vi "Time.Compare New Time with From_To to get new From_To Time Range.vi"(8 "Init":bool, 9 "PrevTo":timestamp, 10 "PrevFrom":timestamp, 11 "Start":timestamp) -> (1 "NewTo":timestamp, 2 "NewFrom":timestamp)   [LabVIEW 2019]
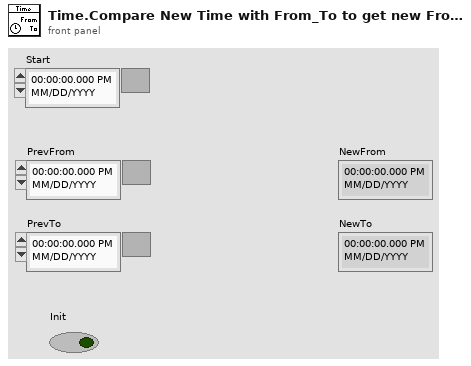
[diagram p1: front panel]
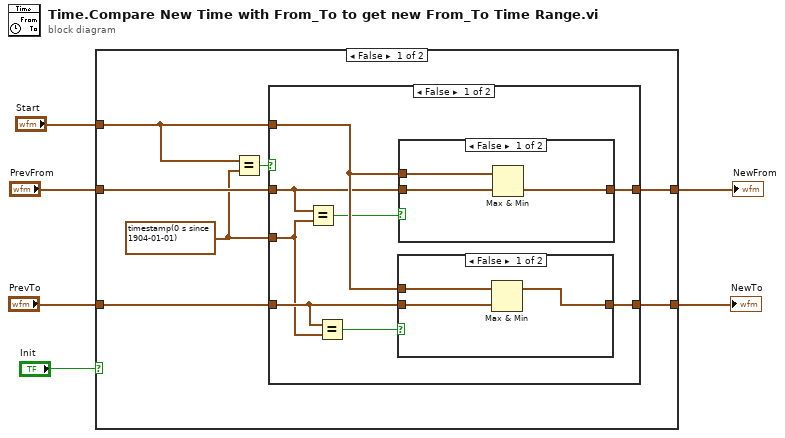
[diagram p0: block diagram]
diagram:
  n1 = case shown="False" "Init" {
    tunnel: "PrevFrom" -> [w13 _]
    tunnel: [w12 w32] -> w5
    tunnel: "Start" -> [w11 w32]
    tunnel: "PrevTo" -> [w9 _]
    tunnel: [w7 w32] -> w2
    frame False {
      w8 = timestamp(0 s since 1904-01-01)
      n2 = Equal?(x=w11, y=w8) -> (x = y?=w10:bool)
      n3 = case shown="False" w10 {
        tunnel: w13 -> [w16 w31]
        tunnel: [w21 w31] -> w12
        tunnel: w11 -> [w20 _]
        tunnel: w9 -> [w18 w30]
        tunnel: w8 -> [w15 _]
        tunnel: [w14 w30] -> w7
        frame False {
          n4 = Equal?(x=w16, y=w15) -> (x = y?=w17:bool)
          n5 = Equal?(x=w18, y=w15) -> (x = y?=w19:bool)
          n6 = case shown="False" w19 {
            tunnel: w20 -> [w24 w25]
            tunnel: w18 -> [w23 _]
            tunnel: [w22 w25] -> w14
            frame False {
              n7 = Max & Min(x=w24, y=w23) -> (max(x,y)=w22:timestamp)  [unwired: 1 out]
            }
            frame True {
            }
          }
          n8 = case shown="False" w17 {
            tunnel: w20 -> [w28 w29]
            tunnel: w16 -> [w27 _]
            tunnel: [w26 w29] -> w21
            frame False {
              n9 = Max & Min(x=w28, y=w27) -> (min(x,y)=w26:timestamp)  [unwired: 1 out]
            }
            frame True {
            }
          }
        }
        frame True {
        }
      }
    }
    frame True {
    }
  }
  "NewFrom" <- w5
  "NewTo" <- w2
